vi "Get Parity Bit.vi"(11 "Array in":bool[](array[boolean])) -> (2 "Parity Bit":bool, 3 "Array out":bool[](array[boolean]))   [LabVIEW 2023]
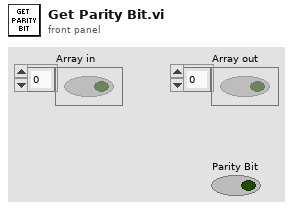
[diagram p1: front panel]
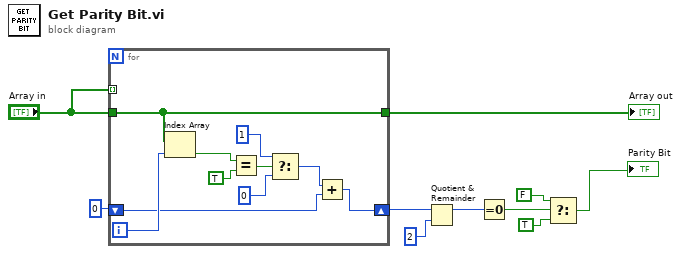
[diagram p0: block diagram]
diagram:
  n1 = for {
    tunnel: "Array in" -> [_] mode=indexing
    tunnel: "Array in" -> [w11]
    shift-right: [w13] -> w3
    shift-left: u16 0 -> [w12]
    tunnel: [w11] -> w9
    i -> [w20]
    n2 = Index Array(array=w11, index=w20) -> (element=w19:bool)
    n3 = Equal?(x=w19, y=TRUE) -> (x = y?=w16:bool)
    n4 = Select(t=u16 1, s=w16, f=u16 0 ("t")) -> (s? t:f=w17:u16)
    n5 = Add(x=w17, y=w12) -> (x+y=w13:u16)
  }
  "Array out" <- w9
  n6 = Quotient & Remainder(x=w3, y=u16 2) -> (x-y*floor(x/y)=w5:u16)  [unwired: 1 out]
  n7 = Equal To 0?(x=w5) -> (x = 0?=w6:bool)
  n8 = Select(t=FALSE, s=w6, f=TRUE) -> (s? t:f=→"Parity Bit":bool)
